vi "Remove MC sections and keys.vi"(11 "User profile ref":T1) -> (3 "User profile ref":T1)   [LabVIEW 2017]
uses:
  <vilib>/Utility/config.llb/Config Data RefNum.ctl
  <vilib>/Utility/config.llb/NI_LVConfig.lvlib
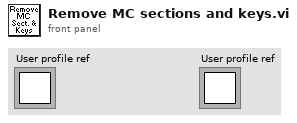
[diagram p1: front panel]
types:
  T1 = typedef "NI_LVConfig.lvlib/Config Data RefNum.ctl" = refnum<k1>
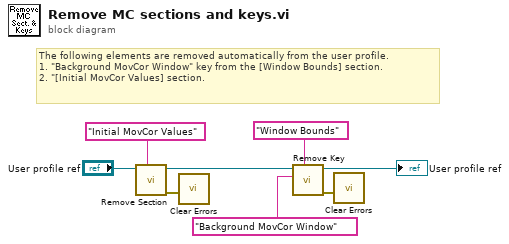
[diagram p0: block diagram]
diagram:
  # "The following elements are removed automatically from the user profile.\n1.\t\"Background MovCor Window\" key from the [Window Bounds] section.\n2.\t\"[Initial MovCor Values] section."
  n1 = call <vilib>:"Remove Section.vi"("section"="Initial MovCor Values", "refnum"="User profile ref") -> ("error out"=w3:errorcluster, "refnum out"=w5:T1)  [unwired: 7 in, 1 out]
  n2 = call <vilib>:"Clear Errors.vi"("error in (no error)"=w3) -> ()  [unwired: 5 in, 2 out]
  n3 = call <vilib>:"Remove Key.vi"("section"="Window Bounds", "key"="Background MovCor Window", "refnum"=w5) -> ("error out"=w6:errorcluster, "refnum out"=→"User profile ref":T1)  [unwired: 6 in, 1 out]
  n4 = call <vilib>:"Clear Errors.vi"("error in (no error)"=w6) -> ()  [unwired: 5 in, 2 out]
